vi "irrad calc duv.vi"(8 "error in (no error)":errorcluster, 10 "IRRAD Input Parameters":T1, 11 "Color Parameters in":T2) -> (0 "error out":errorcluster, 2 "IRRAD Input Parameters out":T1, 3 "Color Parameters out":T2)   [LabVIEW 2013, in "AvaSpec.lvlib" / "AVSirrad_support.lvlib"]
uses:
  AVSirrad_support.lvlib
  Acquisition/AvaSpec Color Parameters.ctl
  IRRAD input parameters.ctl
  <vilib>/Analysis/polynomials.llb/Scalar Polynomial Evaluation (DBL).vi
  <vilib>/express/express arith-compare/Formula/XNode/ExpressFormulaBlockNode.xnode
  <vilib>/Analysis/NI_AALPro.lvlib
  AvaSpec.lvlib
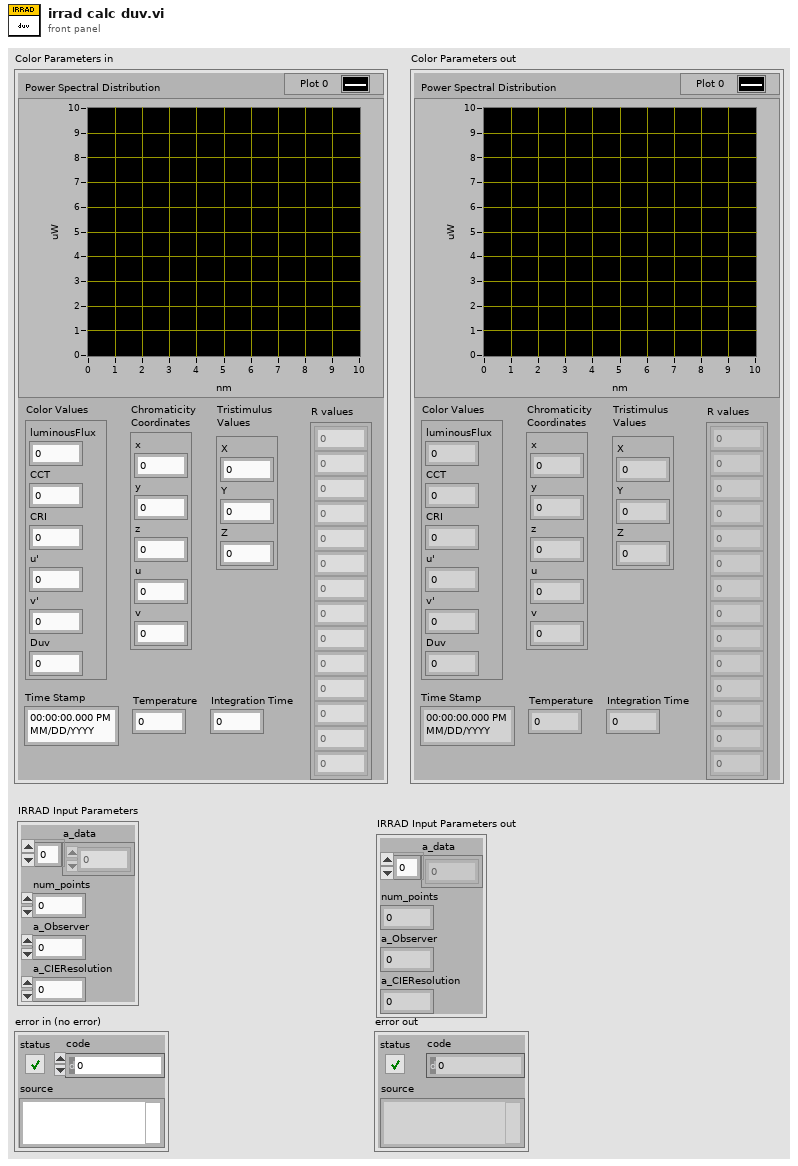
[diagram p1: front panel]
types:
  T1 = typedef "IRRAD input parameters.ctl" = cluster{"a_data":dbl[], "num_points":i32, "a_Observer":u8, "a_CIEResolution":u8}
  T2 = typedef "AvaSpec.lvlib/AvaSpec Color Parameters.ctl" = cluster{"Power Spectral Distribution":cluster{"X":dbl, "Y":dbl}[], "Color Values":cluster{"luminousFlux":dbl, "CCT":dbl, "CRI":dbl, "u'":dbl, "v'":dbl, "Duv":dbl}, "R values":dbl[], "Chromaticity \nCoordinates":cluster{"x":dbl, "y":dbl, "z":dbl, "u":dbl, "v":dbl}, "Tristimulus \nValues":cluster{"X":dbl, "Y":dbl, "Z":dbl}, "Time Stamp":timestamp, "Temperature":dbl, "Integration Time":dbl}
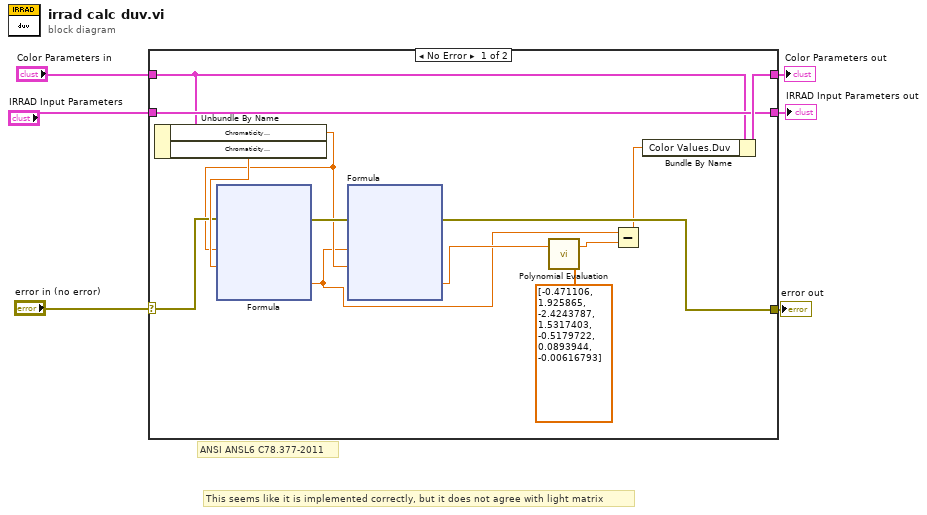
[diagram p0: block diagram]
diagram:
  # "This seems like it is implemented correctly, but it does not agree with light matrix"
  # "ANSI ANSL6 C78.377-2011"
  n1 = case shown="No Error" "error in (no error)" {
    selector: "error in (no error)" -> [w12 w42]
    tunnel: [w11 w42] -> w2
    tunnel: "Color Parameters in" -> [w17 w41]
    tunnel: [w19 w41] -> w4
    tunnel: "IRRAD Input Parameters" -> [w18 w40]
    tunnel: [w18 w40] -> w6
    frame No Error {
      n2 = Unbundle By Name(w17) -> ("Chromaticity \nCoordinates.u"=w8:dbl, "Chromaticity \nCoordinates.v"=w16:dbl)
      n3 = xnode "Formula"("u"=w8, "v"=w16, "error in (no error)"=w12) -> ("Result"=w7:dbl, "error out"=w13:errorcluster)
      n4 = xnode "Formula"("Lfp"=w7, "u"=w8, "error in (no error)"=w13) -> ("Result"=w14:dbl, "error out"=w11:errorcluster)
      n5 = call-poly <vilib>:"Polynomial Evaluation.vi"("P(x)"=dbl[] [-0.471106, 1.925865, -2.4243787, 1.5317403, -0.5179722, 0.0893944, -0.00616793] ("reversed array"), "a"=w14) -> ("P(a)"=w15:dbl)  [unwired: 1 out]
      n6 = Subtract(x=w7, y=w15) -> (x-y=w10:dbl)
      n7 = Bundle By Name(cluster=w17, "Color Values.Duv"=w10) -> (w19:T2)
    }
    frame Error {
    }
  }
  "error out" <- w2
  "Color Parameters out" <- w4
  "IRRAD Input Parameters out" <- w6
